vi "setPermissions.vi"(8 "error in (no error)":errorcluster, 11 "FileTransfer in":refnum<class "FileTransfer.lvclass">) -> (0 "error out":errorcluster, 3 "FileTransfer out":refnum<class "FileTransfer.lvclass">)   [LabVIEW 2016, in "FileTransfer.lvclass"]
uses:
  FileTransfer.lvclass
  FileTransfer.lvclass/FileTransfer.ctl
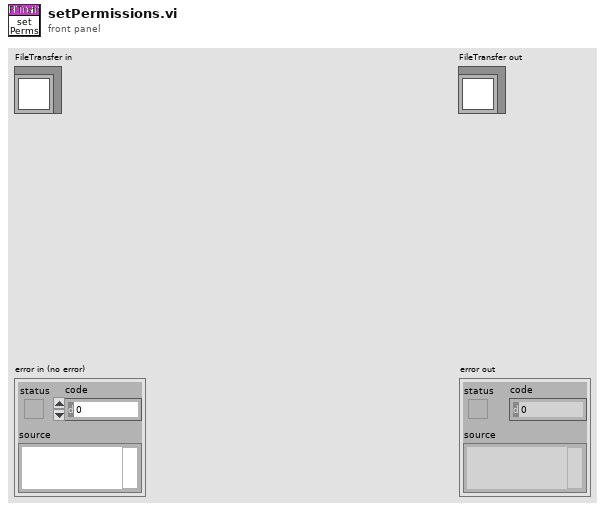
[diagram p1: front panel]
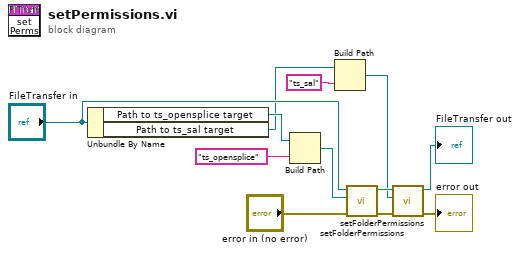
[diagram p0: block diagram]
diagram:
  n1 = Unbundle By Name("FileTransfer in") -> ("Path to ts_opensplice target"=w6:path, "Path to ts_sal target"=w4:path)
  n2 = Build Path(base path=w6, name or relative path="ts_opensplice" ("spreadsheet string")) -> (appended path=w1:path)
  n3 = Build Path(base path=w4, name or relative path="ts_sal" ("spreadsheet string")) -> (appended path=w2:path)
  n4 = call "setFolderPermissions.vi"("error in (no error)"="error in (no error)", "folderPath"=w1, "FileTransfer in"="FileTransfer in") -> ("error out"=w11:errorcluster, "FileTransfer out"=w12:refnum<class "FileTransfer.lvclass">)  [unwired: 7 in]
  n5 = call "setFolderPermissions.vi"("error in (no error)"=w11, "folderPath"=w2, "FileTransfer in"=w12) -> ("error out"=→"error out":errorcluster, "FileTransfer out"=→"FileTransfer out":refnum<class "FileTransfer.lvclass">)  [unwired: 7 in]
